vi "控件颜色变更.vi"(7 "更新":bool=TRUE, 8 "error in (no error)":errorcluster caption="错误输入（无错误）", 9 "控件选择":enum16{"自动", "手动", "设置", "校准", "退出"}(ring), 10 "选项":enum16{"控件引用获取", "设置属性背景色", "还原所有背景色"}(ring), 11 "引用":refnum<vi>[](array[refnum])) -> (0 "error out":errorcluster caption="错误输出", 3 "控件":i32)   [LabVIEW 2014]
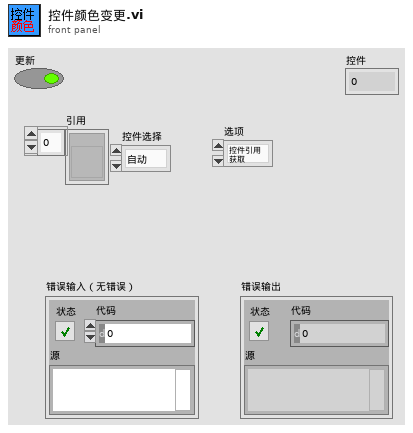
[diagram p1: front panel]
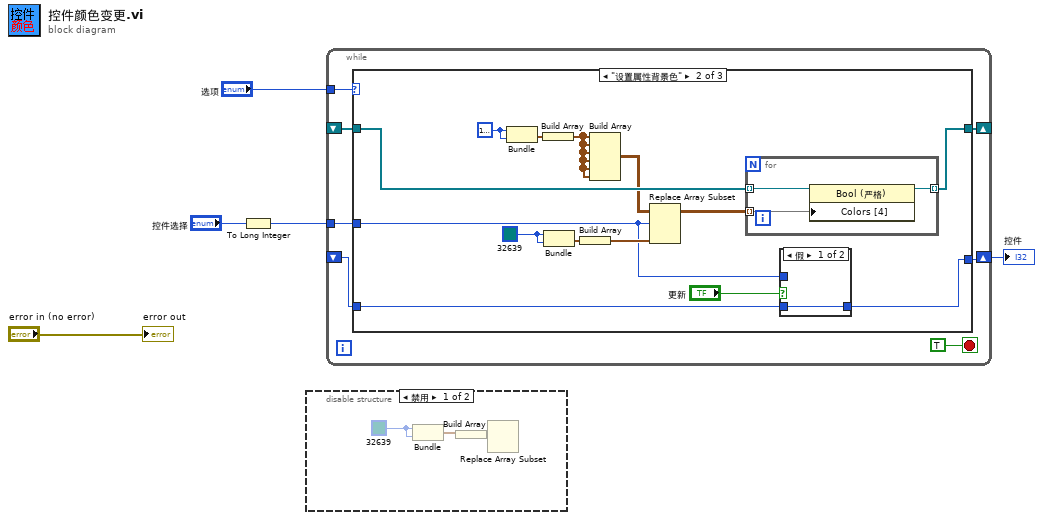
[diagram p0: block diagram]
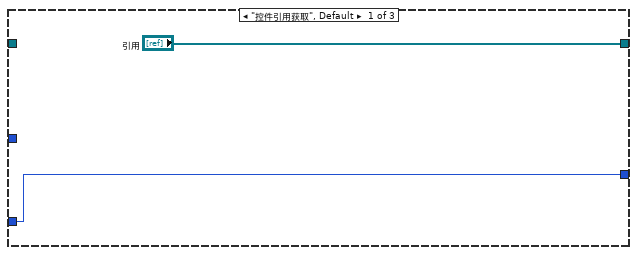
[diagram p3: hidden frame]
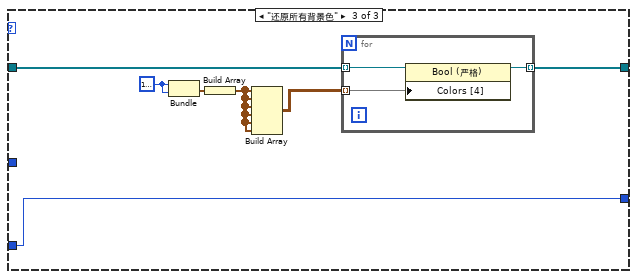
[diagram p5: hidden frame]
diagram:
  n1 = To Long Integer(number="控件选择") -> (32bit integer=w3:i32)
  n2 = disable-structure shown="禁用" {
    frame Disabled {
      w8 = u32 32639
      n3 = Bundle(w8, w8) -> (w7:cluster{u32, u32})  [unwired: 1 in]
      n4 = Build Array(w7) -> (w9:cluster{u32, u32}[])
      n5 = Replace Array Subset() -> (index=w6:i32)  [unwired: 2 in, 1 out]
    }
    frame Enabled {
    }
  }
  n6 = while {
    tunnel: "选项" -> [w15]
    shift-right: [w14] -> _
    shift-left: _ -> [w13]
    tunnel: w3 -> [w12]
    shift-right: [w11] -> w1
    shift-left: _ -> [w10]
    stop <- TRUE stop-if-true
    n7 = case shown="\"设置属性背景色\"" w15 {
      tunnel: ["引用" w31 w43] -> w14
      tunnel: w13 -> [_ w32 w44]
      tunnel: w12 -> [_ w21 _]
      tunnel: [w17 w20 w38] -> w11
      tunnel: w10 -> [w17 w19 w38]
      frame "控件引用获取", Default {
      }
      frame "设置属性背景色" {
        w26 = u32 32639
        w30 = u32 16777216
        n8 = Bundle(w30, w30) -> (w29:cluster{u32, u32})  [unwired: 1 in]
        n9 = Build Array(w29) -> (w24:cluster{u32, u32}[])
        n10 = Bundle(w26, w26) -> (w27:cluster{u32, u32})  [unwired: 1 in]
        n11 = Build Array(w27) -> (w25:cluster{u32, u32}[])
        n12 = Build Array(w24, w24, w24, w24, w24, w24) -> (w28:cluster{u32, u32}[][])
        n13 = Replace Array Subset(array=w28, new element=w25, index (row)=w21) -> (w23:cluster{u32, u32}[][])  [unwired: 1 in]
        n14 = for {
          tunnel: w32 -> [w37] mode=indexing
          tunnel: [w36] -> w31 mode=indexing
          tunnel: w23 -> [w35] mode=indexing
          n15 = property class="Bool (严格)"(reference=w37, "Colors [4]"=w35) -> (reference out=w36:refnum<vi>)  [unwired: 1 in, 1 out]
        }
        n16 = case shown="假" "更新" {
          tunnel: w21 -> [_ w34]
          tunnel: [w33 w34] -> w20
          tunnel: w19 -> [w33 _]
          frame False {
          }
          frame True {
          }
        }
      }
      frame "还原所有背景色" {
        w42 = u32 16777216
        n17 = Bundle(w42, w42) -> (w41:cluster{u32, u32})  [unwired: 1 in]
        n18 = Build Array(w41) -> (w40:cluster{u32, u32}[])
        n19 = Build Array(w40, w40, w40, w40, w40, w40) -> (w39:cluster{u32, u32}[][])
        n20 = for {
          tunnel: w44 -> [w47] mode=indexing
          tunnel: [w46] -> w43 mode=indexing
          tunnel: w39 -> [w45] mode=indexing
          n21 = property class="Bool (严格)"(reference=w47, "Colors [4]"=w45) -> (reference out=w46:refnum<vi>)  [unwired: 1 in, 1 out]
        }
      }
    }
  }
  "控件" <- w1
  "error out" <- "error in (no error)"
